vi "MAIN_SALICRU_API_EMS.vi"() -> ()   [LabVIEW 2024]
uses:
  SALICRUAPI.lvlib
panel:
  out "Consumo total":dbl
  out "red":dbl
  out "Inverter":dbl
  out "error out":errorcluster
  in  "stop":bool
  out "Values":map{string, dbl}(c390)
  out "Inverter alarms":i32[](array[numeric])
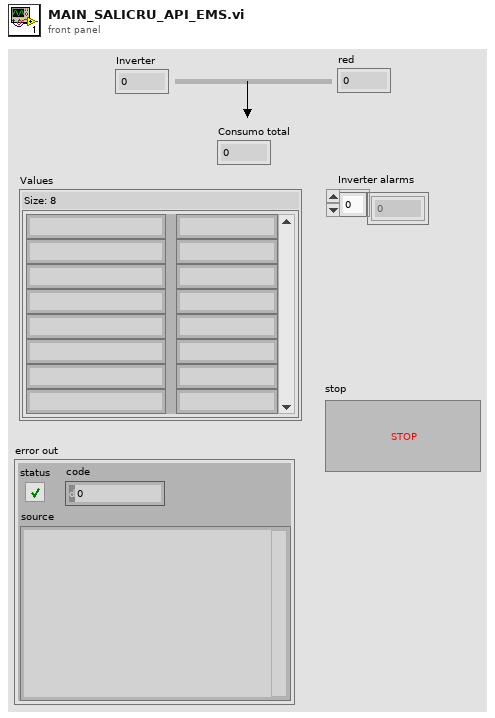
[diagram p1: front panel]
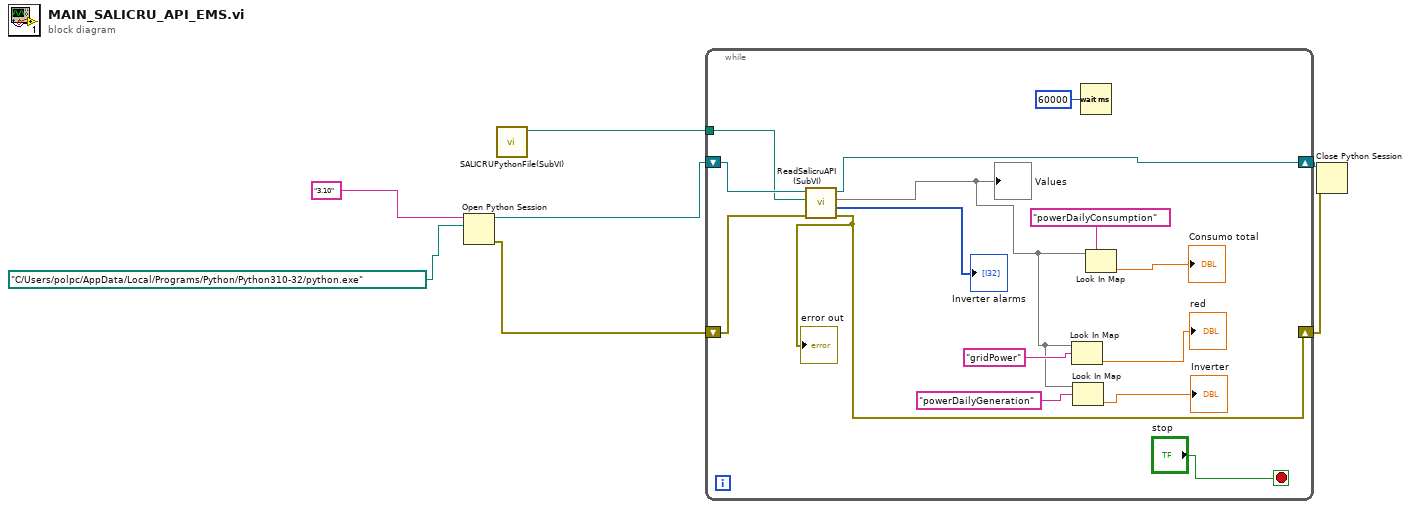
[diagram p0: block diagram]
diagram:
  n1 = Open Python Session(python version="3.10" ("Python version"), python path=path "C:/Users/polpc/AppData/Local/Programs/Python/Python310-32/python.exe") -> (session out=w2:refnum<k35>, error out=w1:errorcluster)  [unwired: 1 in]
  n2 = call "SALICRUPythonFile(SubVI).vi"() -> ("SALICRU WRAPPER FILE"=w3:path)  [unwired: 11 in]
  n3 = while {
    shift-right: [w22] -> w5
    shift-left: w2 -> [w20]
    shift-right: [w21] -> w4
    shift-left: w1 -> [w19]
    tunnel: w3 -> [w17]
    stop <- "stop" stop-if-true
    n4 = call "ReadSalicruAPI (SubVI).vi"("error in (no error)"=w19, "Python File"=w17, "session in"=w20) -> ("error out"=w21:errorcluster, "Array"=→"Inverter alarms":i32[], "Map"=w11:map{string, dbl}, "session out"=w22:refnum<k35>)  [unwired: 5 in]
    "Values" <- w11
    "error out" <- w21
    n5 = Look In Map(map=w11, key="gridPower") -> (value=→"red":dbl)  [unwired: 1 in, 1 out]
    n6 = Look In Map(map=w11, key="powerDailyGeneration") -> (value=→"Inverter":dbl)  [unwired: 1 in, 1 out]
    n7 = Wait (ms)(milliseconds to wait=u32 60000) -> ()  [unwired: 1 out]
    n8 = Look In Map(map=w11, key="powerDailyConsumption") -> (value=→"Consumo total":dbl)  [unwired: 1 in, 1 out]
  }
  n9 = Close Python Session(session in=w5, error in=w4) -> ()  [unwired: 1 out]
